vi "Initialize.vi"(8 "error in (no error)":errorcluster, 10 "ctrl":refnum<vi>, 11 "IB_Tree in":refnum<class "IB_Tree.lvclass">) -> (0 "error out":errorcluster, 3 "IB_Tree out":refnum<class "IB_Tree.lvclass">)   [LabVIEW 2020, in "IB_Tree.lvclass"]
uses:
  <vilib>/AppBuilder/IB_Classes/Tree/IB_Tree.lvclass
  <vilib>/AppBuilder/IB_Classes/Tree/IB_Tree.lvclass/IB_Tree.ctl
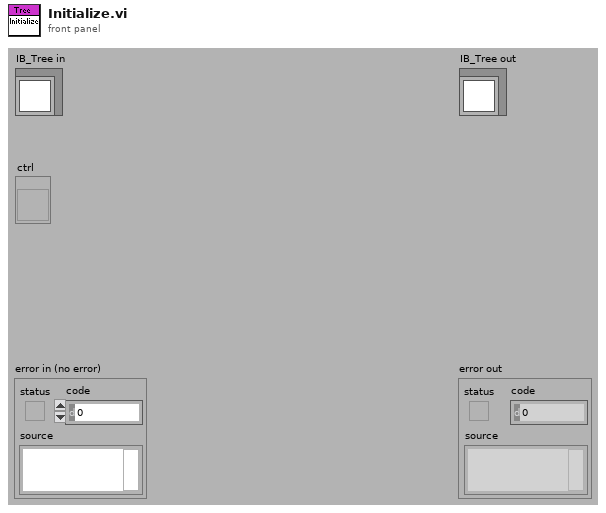
[diagram p1: front panel]
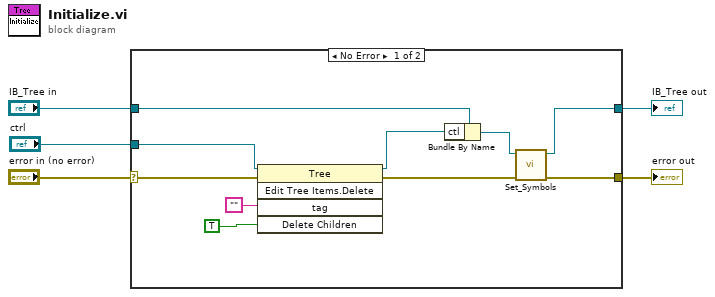
[diagram p0: block diagram]
diagram:
  n1 = case shown="No Error" "error in (no error)" {
    selector: "error in (no error)" -> [w13 w17]
    tunnel: [w8 w17] -> w4
    tunnel: [w6 w16] -> w2
    tunnel: "IB_Tree in" -> [w11 w16]
    tunnel: "ctrl" -> [w12 _]
    frame No Error {
      n2 = invoke class="Tree" method="Edit Tree Items.Delete"(reference=w12, error in=w13, "tag"="", "Delete Children"=TRUE ("Delete Children?")) -> (reference out=w10:refnum<vi>, error out=w9:errorcluster)  [unwired: 1 in, 3 out]
      n3 = Bundle By Name(cluster=w11, "ctl"=w10) -> (w7:refnum<class "IB_Tree.lvclass">)
      n4 = call <vilib>:"Set_Symbols.vi"("error in (no error)"=w9, "IB_Tree in"=w7) -> ("error out"=w8:errorcluster, "IB_Tree out"=w6:refnum<class "IB_Tree.lvclass">)  [unwired: 8 in]
    }
    frame Error {
    }
  }
  "error out" <- w4
  "IB_Tree out" <- w2
